vi "VIPM Uninstall VI Packages By Name.vi"   [LabVIEW 2016, in "Script.lvlib"]
uses:
  Script.lvlib
  <vilib>/Wiresmith Technology/G CLI/Argument Parser/Option Class/Option Configuration.ctl
  <vilib>/Wiresmith Technology/G CLI/Argument Parser/Option Class/Argument Type.ctl
  <vilib>/Wiresmith Technology/G CLI/CLI Class/CLI.lvclass
  <vilib>/Wiresmith Technology/G CLI/Argument Parser/Option Class/Option.lvclass
  <vilib>/Wiresmith Technology/G CLI/Argument Parser/Option Set Class/Option Set.lvclass
  <vilib>/JKI/VIPM API/VIPM API_vipm_api.lvlib
types:
  T1 = typedef "Option Parser.lvlib/Option.lvclass/Option Configuration.ctl" = cluster{"Option Type":T2, "Option Labels":string[], "Key":string, "Description":string, "Required":bool, "Default Value":string}
  T2 = typedef "Option Parser.lvlib/Option.lvclass/Argument Type.ctl" = enum16{"flag", "value"}
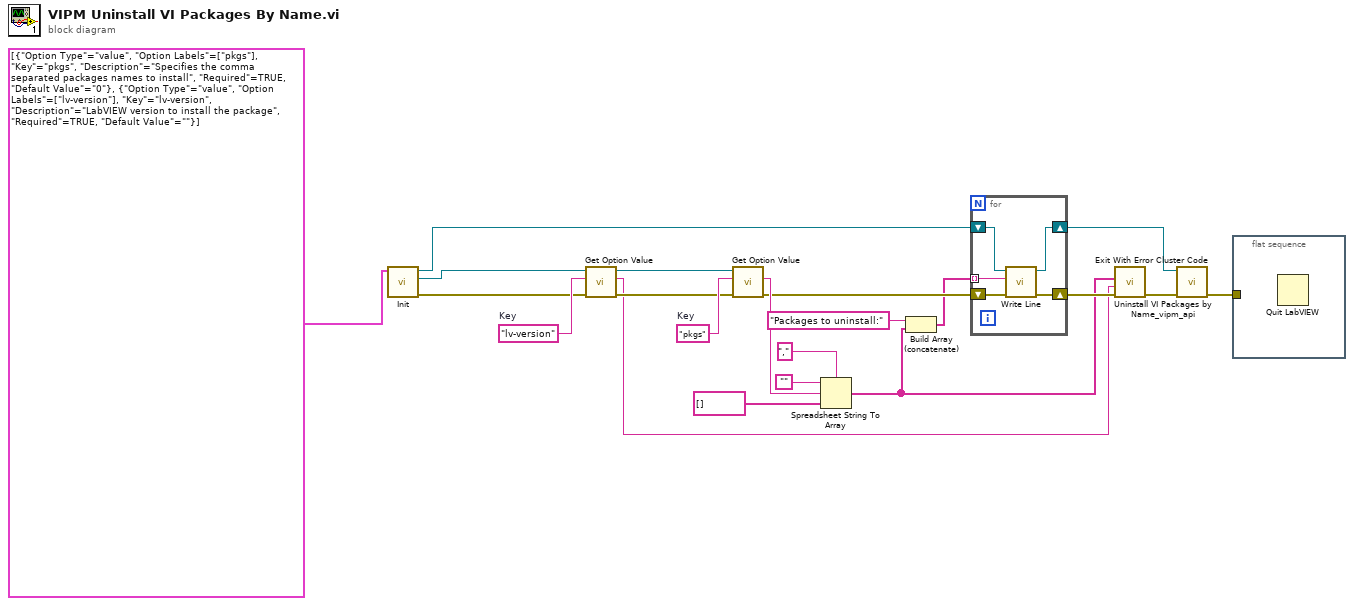
[diagram p0: block diagram]
diagram:
  w14 = "lv-version"  # Key
  w21 = "pkgs"  # Key
  n1 = call "Init.vi"("Options"=T1[] [{"Option Type"=enum."value", "Option Labels"=["pkgs"], "Key"="pkgs", "Description"="Specifies the comma separated packages names to install", "Required"=TRUE, "Default Value"="0"}, {"Option Type"=enum."value", "Option Labels"=["lv-version"], "Key"="lv-version", "Description"="LabVIEW version to install the package", "Required"=TRUE, "Default Value"=""}]) -> ("error out"=w4:errorcluster, "Option Set out"=w3:refnum<class "Option Set.lvclass">, "CLI out"=w2:refnum<class "CLI.lvclass">)  [unwired: 8 in]
  n2 = call <vilib>:"Get Option Value.vi"("error in (no error)"=w4, "Option Key"=w14, "Option Set in"=w3) -> ("error out"=w13:errorcluster, "Value"=w11:string, "Option Set out"=w12:refnum<class "Option Set.lvclass">)  [unwired: 5 in, 1 out]
  n3 = call <vilib>:"Get Option Value.vi"("error in (no error)"=w13, "Option Key"=w21, "Option Set in"=w12) -> ("error out"=w8:errorcluster, "Value"=w10:string)  [unwired: 5 in, 2 out]
  n4 = Spreadsheet String To Array(delimiter (Tab)=",", format string="", spreadsheet string=w10, array type (2D Dbl)=string[] [] ("Value")) -> (array=w6:string[])
  n5 = Build Array (concatenate)("Packages to uninstall:" ("delimiter (Tab)"), w6) -> (w5:string[])
  n6 = for {
    shift-right: [w24] -> w17
    shift-left: w2 -> [w26]
    shift-right: [w25] -> w19
    shift-left: w8 -> [w23]
    tunnel: w5 -> [w22] mode=indexing
    n7 = call <vilib>:"Write Line.vi"("error in (no error)"=w23, "Text to Write"=w22, "CLI in"=w26) -> ("error out"=w25:errorcluster, "CLI out"=w24:refnum<class "CLI.lvclass">)  [unwired: 7 in]
  }
  n8 = call <vilib>:"Uninstall VI Packages by Name_vipm_api.vi"("error in (no error)"=w19, "LabVIEW Version"=w11, "Package Names to Uninstall []"=w6) -> ("error out"=w18:errorcluster)  [unwired: 8 in]
  n9 = call <vilib>:"Exit With Error Cluster Code.vi"("error in (no error)"=w18, "CLI in"=w17) -> ("error out"=w20:errorcluster)  [unwired: 9 in]
  n10 = flat-sequence {
    tunnel: w20 -> [_]
    frame #0 {
      n11 = Quit LabVIEW() -> ()  [unwired: 1 in]
    }
  }
